vi "arm pid.vi"(1 "Setpoint":dbl, 2 "Autotune?":bool) -> (0 "Output":dbl)   [LabVIEW 2013]
uses:
  <vilib>/addons/control/pid/pid.llb/PID (DBL).vi
  <vilib>/addons/control/pid/NI_PID_autopid.lvlib
  <vilib>/addons/control/pid/NI_PID_pid.lvlib
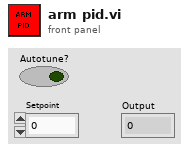
[diagram p1: front panel]
types:
  T1 = cluster{"proportional gain (Kc)":dbl, "integral time (Ti, min)":dbl, "derivative time (Td, min)":dbl}
  T2 = typedef "WPI_EncoderDevRef.ctl" = cluster{"DevStatus":errorcluster, "EncoderIndex":T3, "CounterIndex":T4, "DistancePerCount":dbl, "Decoding Type":T5}
  T3 = typedef "FPGA_EncoderIdx.ctl" = enum8{"Enc 0", "Enc 1", "Enc 2", "Enc 3", "Invalid"}
  T4 = typedef "FPGA_CounterCtrSystemIndex.ctl" = enum8{"Ctr 0", "Ctr 1", "Ctr 2", "Ctr 3", "Ctr 4", "Ctr 5", "Ctr 6", "Ctr 7", "Invalid"}
  T5 = typedef "WPI_EncoderType.ctl" = enum16{"1x", "2x", "4x"}
  T6 = cluster{"controller type":u16, "relay cycles":i32, "relay amplitude":dbl, "control specification":u16, "PV noise level":dbl}
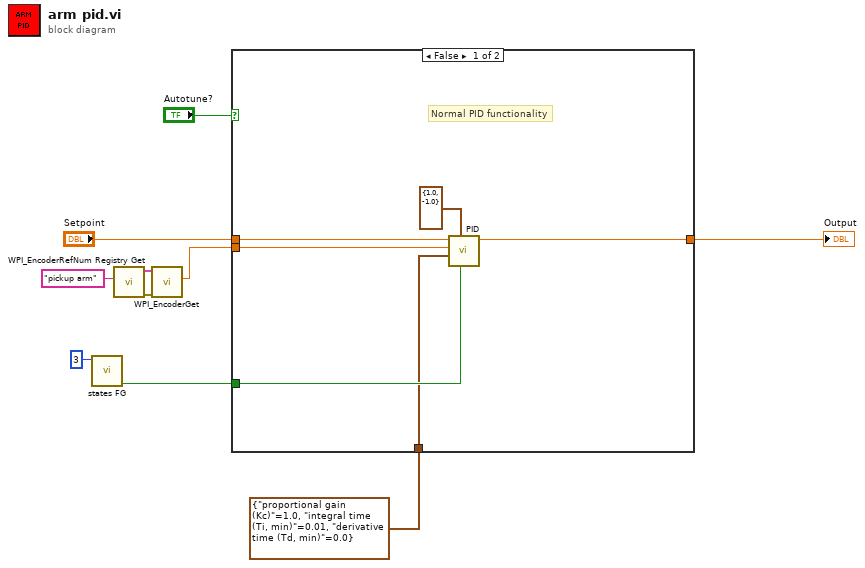
[diagram p0: block diagram]
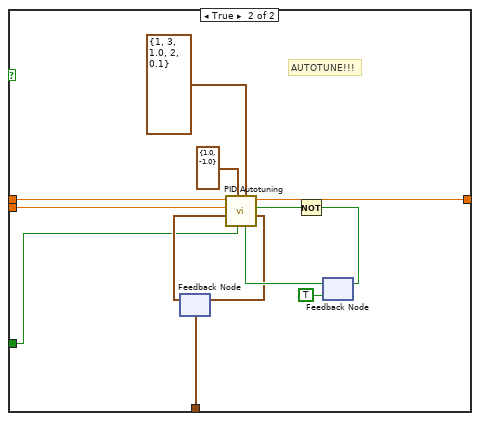
[diagram p2: hidden frame]
diagram:
  n1 = call "states FG.vi"("Loop ID"=3) -> ("first call?"=w2:bool)  [unwired: 7 in, 3 out]
  n2 = call <vilib>:"WPI_EncoderRefNum Registry Get.vi"("refnum name"="pickup arm") -> ("error out"=w8:errorcluster, "EncoderDevRef"=w7:T2)  [unwired: 9 in]
  n3 = call <vilib>:"WPI_EncoderGet.vi"("error in (no error)"=w8, "EncoderDevRef"=w7) -> ("Distance"=w6:dbl)  [unwired: 4 in, 5 out]
  n4 = case shown="False" "Autotune?" {
    tunnel: "Setpoint" -> [w16 w27]
    tunnel: [w15 w26] -> w9
    tunnel: w6 -> [w13 w19]
    tunnel: w2 -> [w14 w18]
    tunnel: T1 {"proportional gain (Kc)"=1.0, "integral time (Ti, min)"=0.01, "derivative time (Td, min)"=0.0} ("PID gains out") -> [w11 w17]
    frame False {
      # "Normal PID functionality"
      n5 = call-poly <vilib>:"PID.vi"("reinitialize? (F)"=w14, "output range"=cluster{"output high":dbl, "output low":dbl} {"output high"=1.0, "output low"=-1.0}, "PID gains"=w11, "process variable"=w13, "setpoint"=w16) -> ("output"=w15:dbl)  [unwired: 5 in, 1 out]
    }
    frame True {
      # "AUTOTUNE!!!"
      n6 = feedback #1(w17) -> (w20:T1)
      n7 = feedback #2(TRUE) -> (w23:bool)
      n8 = call <vilib>:"PID Autotuning.vi"("autotune? (F)"=w23, "autotuning parameters"=T6 {"controller type"=1, "relay cycles"=3, "relay amplitude"=1.0, "control specification"=2, "PV noise level"=0.1}, "reinitialize? (F)"=w18, "output range"=cluster{"output high":dbl, "output low":dbl} {"output high"=1.0, "output low"=-1.0}, "PID gains"=w20, "process variable"=w19, "setpoint"=w27) -> ("PID gains out"=w21:T1, "tuning completed?"=w25:bool, "output"=w26:dbl)  [unwired: 1 in, 1 out]
      n9 = feedback-in #1(w21) -> ()
      n10 = Not(x=w25) -> (.not. x?=w24:bool)
      n11 = feedback-in #2(w24) -> ()
    }
  }
  "Output" <- w9
